vi "example_2_5_c.vi"() -> ()   [LabVIEW 2018]
panel:
  in  "Cluster":T1 {"Knob" scale=0.0..10.0 scale format="%.1f"; "Numeric" format="%.2f"}
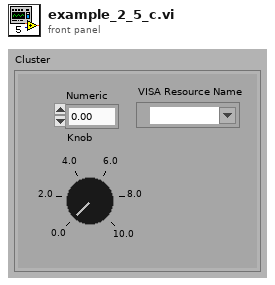
[diagram p1: front panel]
types:
  T1 = cluster{"Numeric":dbl, "Knob":dbl, "VISA Resource Name":refnum<visa-resource-name>}
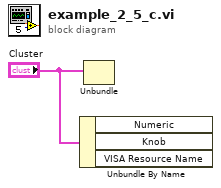
[diagram p0: block diagram]
diagram:
  n1 = Unbundle By Name("Cluster") -> ()  [unwired: 3 out]
  n2 = Unbundle("Cluster") -> ()  [unwired: 3 out]
